vi "simulation3.vi"() -> ()   [LabVIEW 2016]
panel:
  in  "stop":bool
  out "Delta radians":dbl
  out "prev set point dir":dbl(knob) scale=-3.14..3.14
  out "prev set point":i32
  out "Delta ticks":i32
  in  "stop":bool
  out "encoder":i32
  out "backward":bool
  out "forward":bool
  out "Wheel Direction":dbl(knob) scale=-3.14..3.14
  in  "Joystick":dbl(knob) scale=-3.14..3.14
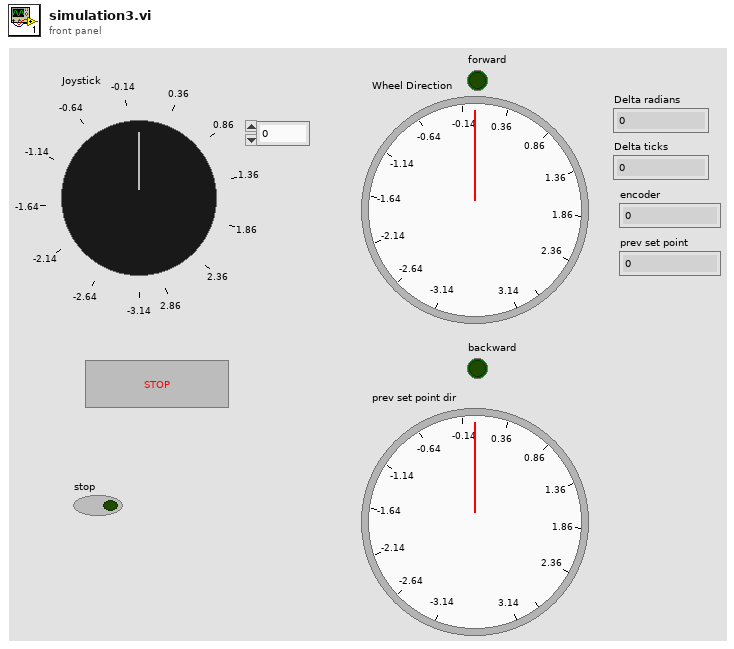
[diagram p1: front panel]
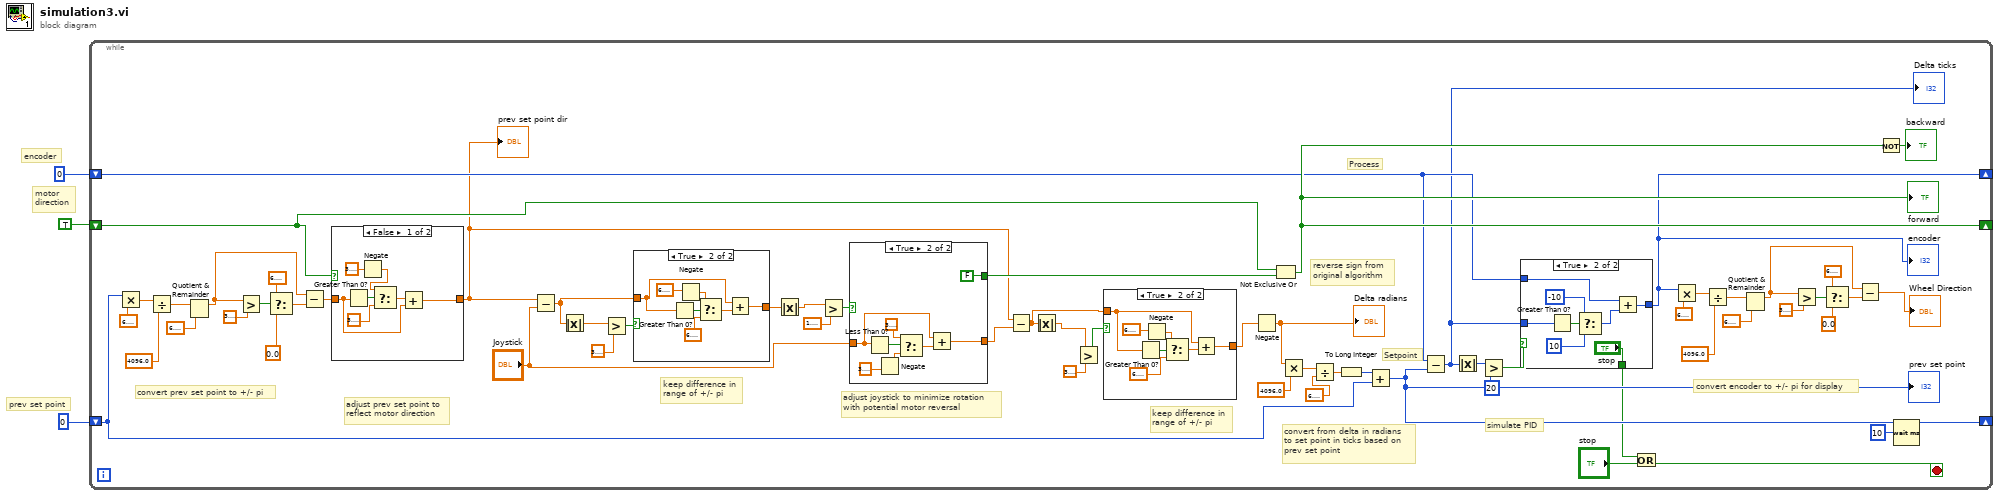
[diagram p0: block diagram]
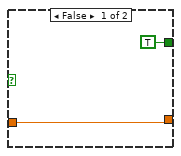
[diagram p3: hidden frame]
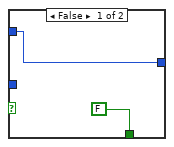
[diagram p6: hidden frame]
diagram:
  # "prev set point"
  # "encoder"
  # "motor\ndirection"
  n1 = while {
    shift-right: [w18] -> _
    shift-left: 0 ("encoder") -> [w35]
    shift-right: [w43] -> _
    shift-left: TRUE -> [w42]
    shift-right: [w34] -> _
    shift-left: 0 ("encoder") -> [w32]
    stop <- w31 stop-if-true
    # "Process"
    # "Setpoint"
    # "keep difference in\nrange of +/- pi"
    # "keep difference in\nrange of +/- pi"
    # "convert from delta in radians\nto set point in ticks based on \nprev set point"
    # "reverse sign from\noriginal algorithm"
    # "convert encoder to +/- pi for display"
    # "adjust prev set point to\nreflect motor direction"
    # "simulate PID"
    # "adjust joystick to minimize rotation\nwith potential motor reversal"
    # "convert prev set point to +/- pi"
    n2 = Multiply(x=w32, y=6.283185307179586) -> (x*y=w62:dbl)
    n3 = Divide(x=w62, y=4096.0) -> (x/y=w60:dbl)
    n4 = Quotient & Remainder(x=w60, y=6.283185307179586) -> (x-y*floor(x/y)=w53:dbl)  [unwired: 1 out]
    n5 = Greater?(x=w53, y=3.141592653589793) -> (0:w57:bool)
    n6 = Select(t=6.283185307179586, s=w57, f=0.0) -> (s? t:f=w54:dbl)
    n7 = Subtract(x=w53, y=w54) -> (x-y=w44:dbl)
    n8 = case shown="False" w42 {
      tunnel: w44 -> [w93 w99]
      tunnel: [w92 w99] -> w16
      frame False {
        n9 = Greater Than 0?(x=w93) -> (x > 0?=w98:bool)
        n10 = Negate(x=3.141592653589793) -> (-x=w97:dbl)
        n11 = Select(t=w97, s=w98, f=3.141592653589793) -> (s? t:f=w94:dbl)
        n12 = Add(x=w94, y=w93) -> (x+y=w92:dbl)
      }
      frame True {
      }
    }
    "prev set point dir" <- w16
    n13 = Subtract(x=w16, y="Joystick") -> (x-y=w13:dbl)
    n14 = Absolute Value(x=w13) -> (abs(x)=w45:dbl)
    n15 = Greater?(x=w45, y=3.141592653589793) -> (0:w14:bool)
    n16 = case shown="True" w14 {
      tunnel: w13 -> [w84 w86]
      tunnel: [w84 w85] -> w12
      frame False {
      }
      frame True {
        n17 = Greater Than 0?(x=w86) -> (x > 0?=w91:bool)
        n18 = Negate(x=6.283185307179586) -> (-x=w88:dbl)
        n19 = Select(t=w88, s=w91, f=6.283185307179586) -> (s? t:f=w87:dbl)
        n20 = Add(x=w86, y=w87) -> (x+y=w85:dbl)
      }
    }
    n21 = Absolute Value(x=w12) -> (abs(x)=w11:dbl)
    n22 = Greater?(x=w11, y=1.5707963267948966) -> (0:w9:bool)
    n23 = case shown="True" w9 {
      tunnel: "Joystick" -> [w74 w78]
      tunnel: [TRUE FALSE] -> w50
      tunnel: [w74 w76] -> w8
      frame False {
      }
      frame True {
        n24 = Less Than 0?(x=w78) -> (x < 0?=w83:bool)
        n25 = Negate(x=3.141592653589793) -> (-x=w80:dbl)
        n26 = Select(t=3.141592653589793, s=w83, f=w80) -> (s? t:f=w79:dbl)
        n27 = Add(x=w78, y=w79) -> (x+y=w76:dbl)
      }
    }
    n28 = Subtract(x=w16, y=w8) -> (x-y=w4:dbl)
    n29 = Absolute Value(x=w4) -> (abs(x)=w6:dbl)
    n30 = Greater?(x=w6, y=3.141592653589793) -> (0:w5:bool)
    n31 = case shown="True" w5 {
      tunnel: w4 -> [w66 w67]
      tunnel: [w66 w68] -> w37
      frame False {
      }
      frame True {
        n32 = Greater Than 0?(x=w67) -> (x > 0?=w73:bool)
        n33 = Negate(x=6.283185307179586) -> (-x=w70:dbl)
        n34 = Select(t=w70, s=w73, f=6.283185307179586) -> (s? t:f=w69:dbl)
        n35 = Add(x=w67, y=w69) -> (x+y=w68:dbl)
      }
    }
    n36 = Negate(x=w37) -> (-x=w15:dbl)
    "Delta radians" <- w15
    n37 = Not Exclusive Or(1:w50, 2:w42) -> (0:w43:bool)
    "forward" <- w43
    n38 = Multiply(x=w15, y=4096.0) -> (x*y=w38:dbl)
    n39 = Divide(x=w38, y=6.283185307179586) -> (x/y=w41:dbl)
    n40 = To Long Integer(number=w41) -> (32bit integer=w36:i32)
    n41 = Add(x=w36, y=w32) -> (x+y=w34:i32)
    "prev set point" <- w34
    n42 = Subtract(x=w35, y=w34) -> (x-y=w33:i32)
    "Delta ticks" <- w33
    n43 = Absolute Value(x=w33) -> (abs(x)=w49:i32)
    n44 = Greater?(x=w49, y=20) -> (0:w47:bool)
    n45 = case shown="True" w47 {
      tunnel: w33 -> [_ w109]
      tunnel: w35 -> [w101 w104]
      tunnel: [w101 w103] -> w18
      tunnel: [FALSE "stop"] -> w30
      frame False {
      }
      frame True {
        n46 = Greater Than 0?(x=w109) -> (x > 0?=w108:bool)
        n47 = Select(t=-10, s=w108, f=10) -> (s? t:f=w105:i32)
        n48 = Add(x=w104, y=w105) -> (x+y=w103:i32)
      }
    }
    "encoder" <- w18
    n49 = Or(x=w30, y="stop") -> (x .or. y?=w31:bool)
    n50 = Multiply(x=w18, y=6.283185307179586) -> (x*y=w28:dbl)
    n51 = Divide(x=w28, y=4096.0) -> (x/y=w26:dbl)
    n52 = Quotient & Remainder(x=w26, y=6.283185307179586) -> (x-y*floor(x/y)=w19:dbl)  [unwired: 1 out]
    n53 = Greater?(x=w19, y=3.141592653589793) -> (0:w23:bool)
    n54 = Select(t=6.283185307179586, s=w23, f=0.0) -> (s? t:f=w20:dbl)
    n55 = Subtract(x=w19, y=w20) -> (x-y=→"Wheel Direction":dbl)
    n56 = Not(x=w43) -> (.not. x?=→"backward":bool)
    n57 = Wait (ms)(milliseconds to wait=u32 10) -> ()  [unwired: 1 out]
  }
